vi "admin tables.vi"() -> ()   [LabVIEW 2020, in "Data.PG.lvclass"]
uses:
  Data.PG.lvclass
panel:
  out "path_to_selected_column":string="llab_038:d001(TEST_TABLE--new_stuff(hippos))"
  in  "Get path":bool
  out "table selected":string
  in  "max characters (if string)":i32
  in  "new column units":string="discoveries"
  in  "new column name":string="successfulness"
  in  "Create Column":bool
  in  "Ring":u16(ring) items=["double", "string", "integer", "boolean"]
  in  "columns_list":i32(listbox)=-1
  in  "new table name":string="TEST_TABLE_2"
  in  "Create Table":bool
  in  "tables_list":i32(listbox)=-1
  in  "STOP":bool
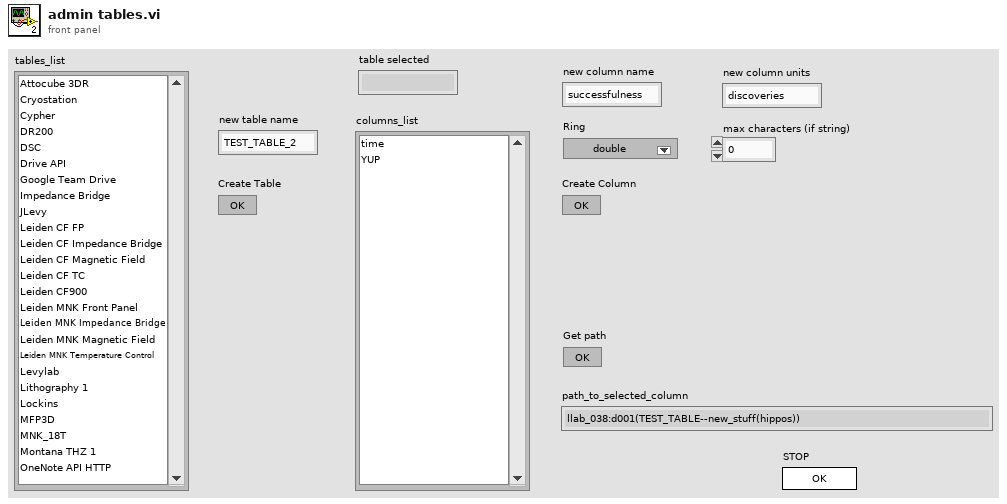
[diagram p1: front panel]
types:
  T1 = enum32{"Invalid", "Standard", "Closed", "Hidden", "Minimized", "Maximized"}
  T2 = enum32{"invalid app kind", "Development System", "Run Time System", "Student Edition", "Embedded LabVIEW", "Evaluation", "Custom"}
  T3 = cluster{"Core":cluster{"Current VI Reference":refnum<vi>, "Close Panel on Exit?":bool}, "Data.PG in":refnum<class "Data.PG.lvclass">, "connection info":cluster{"host":string, "port":string, "dbname":string, "user":string, "password":string}, "table names":string[], "table paths":string[], "column names":string[], "column units":string[], "column paths":string[], "new table name":string, "new column name":string, "new column data type":string, "new column units":string, "selected table":string, "selected column":string, "selected table path":string, "selected column path":string, "Start":timestamp, "End":timestamp, "max points":i32, "selected column units":string}
  T4 = cluster{"host":string, "port":string, "dbname":string, "user":string, "password":string}
  T5 = cluster{"Current VI Reference":refnum<vi>, "Close Panel on Exit?":bool}
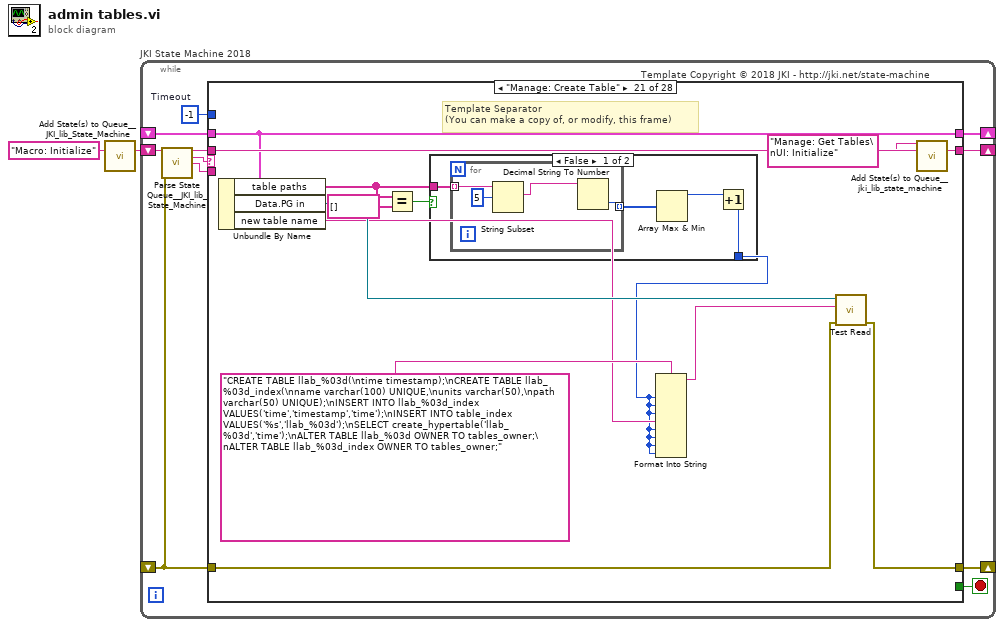
[diagram p0: block diagram]
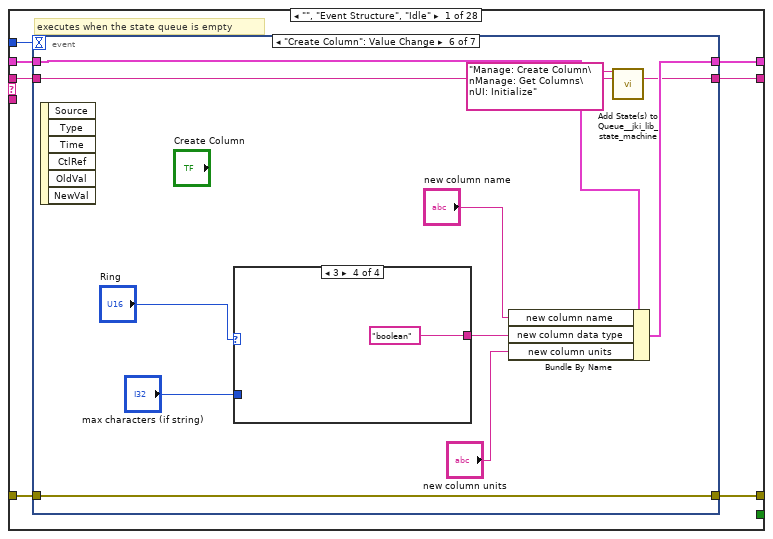
[diagram p2: hidden frame]
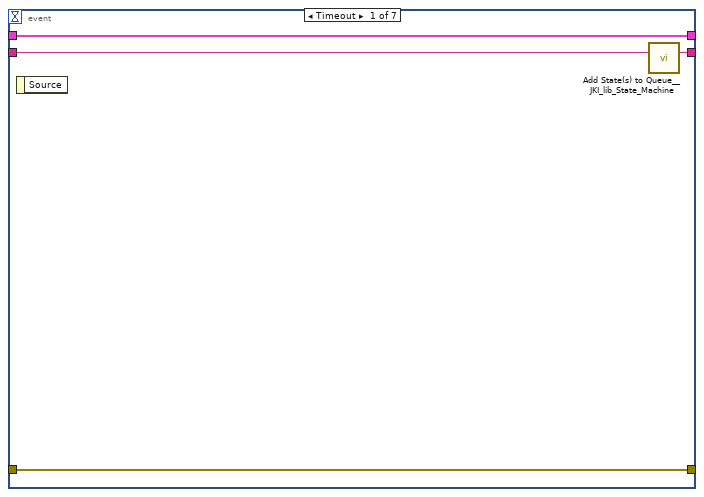
[diagram p3: hidden frame]
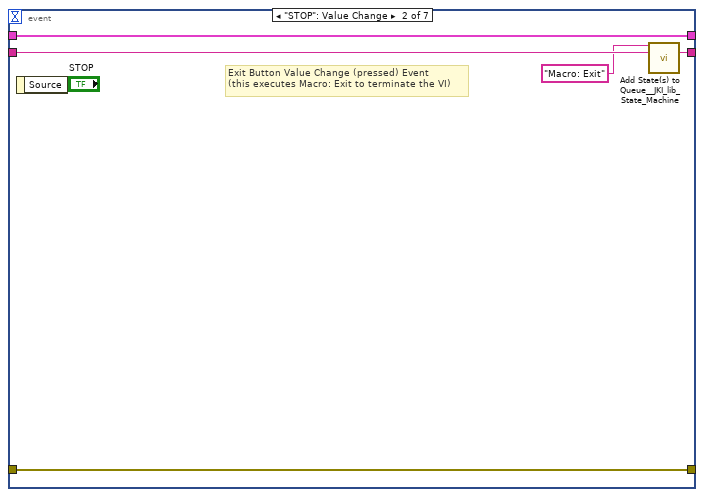
[diagram p4: hidden frame]
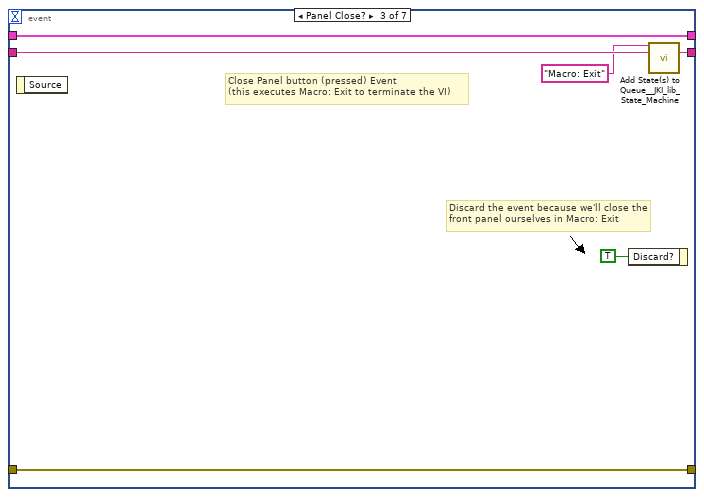
[diagram p5: hidden frame]
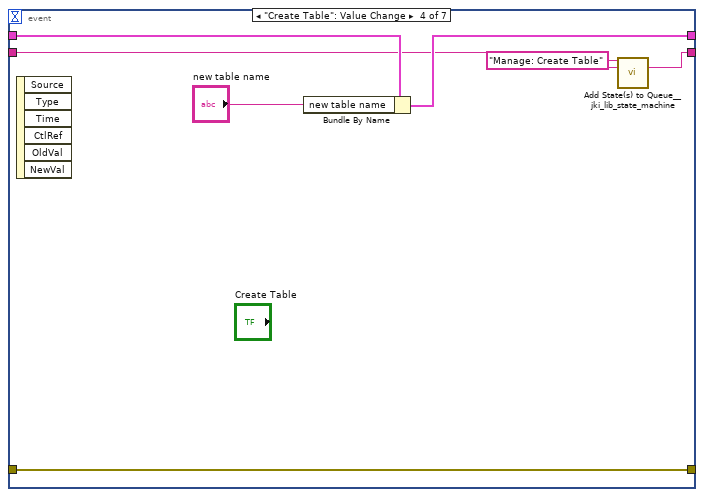
[diagram p6: hidden frame]
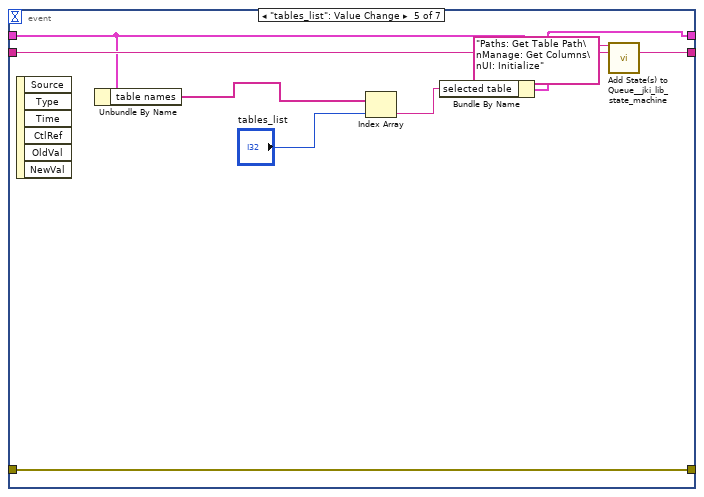
[diagram p7: hidden frame]
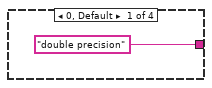
[diagram p8: hidden frame]
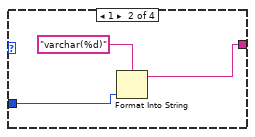
[diagram p9: hidden frame]
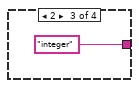
[diagram p10: hidden frame]
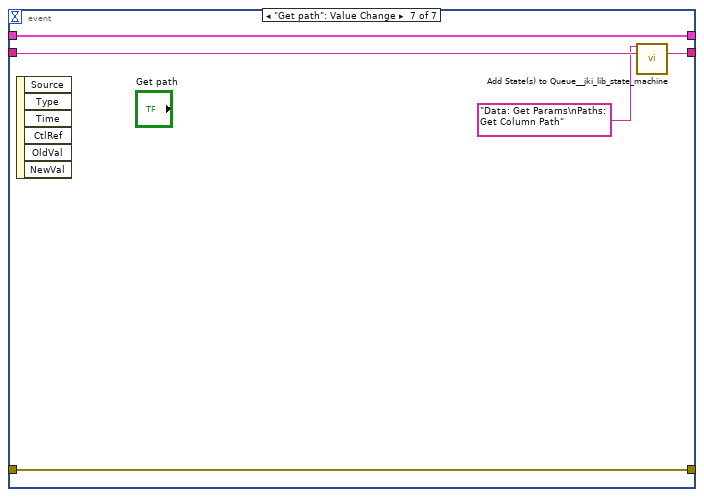
[diagram p11: hidden frame]
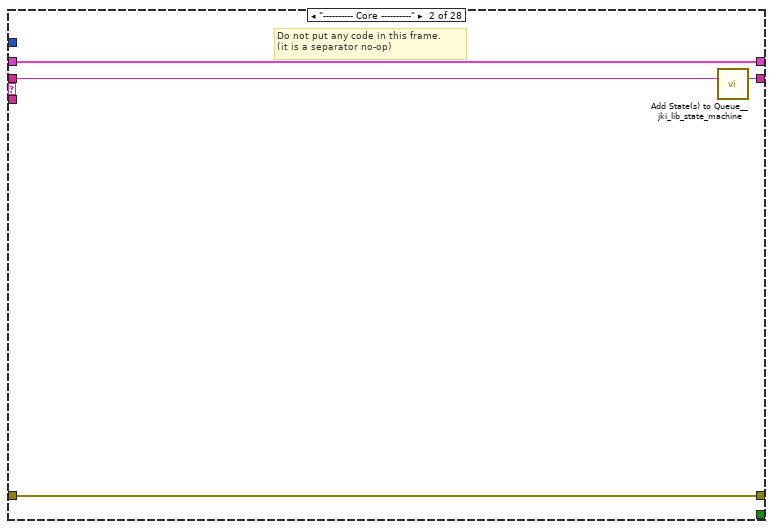
[diagram p12: hidden frame]
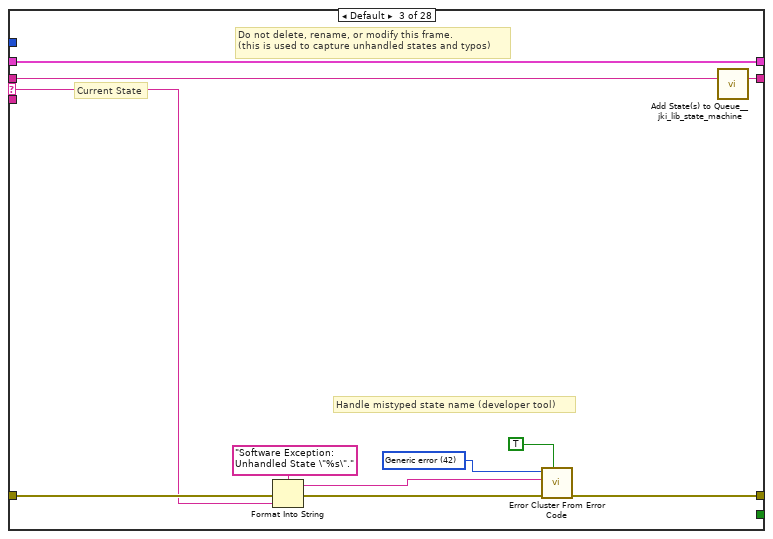
[diagram p13: hidden frame]
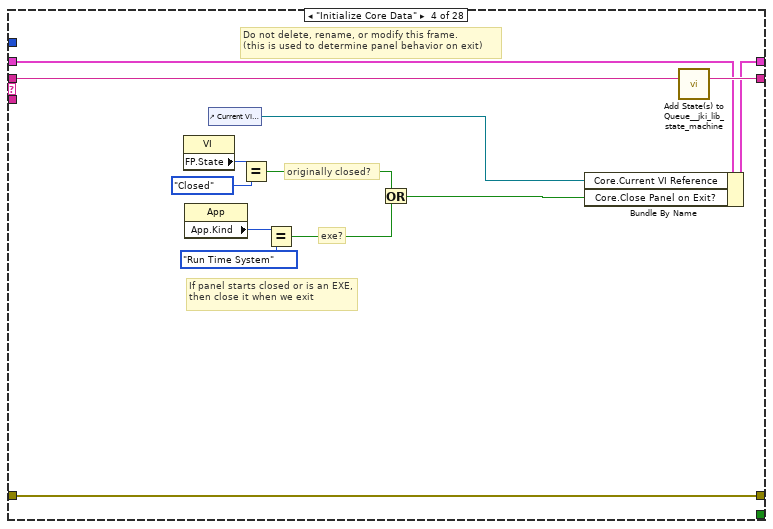
[diagram p14: hidden frame]
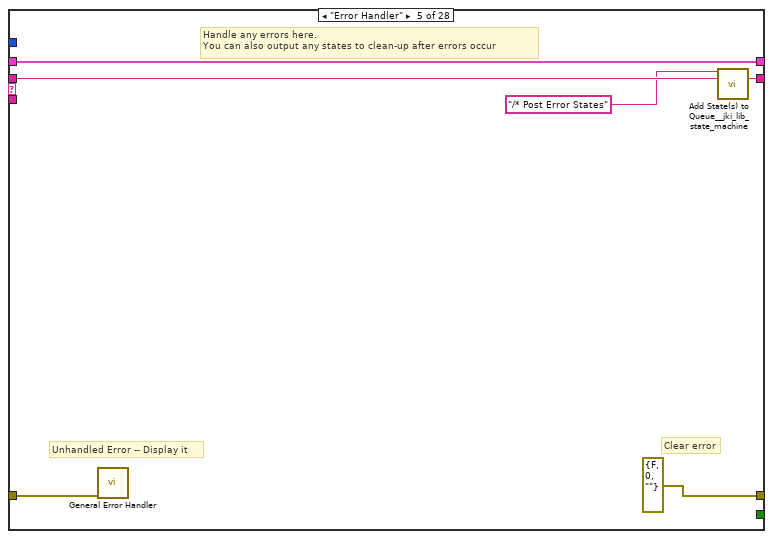
[diagram p15: hidden frame]
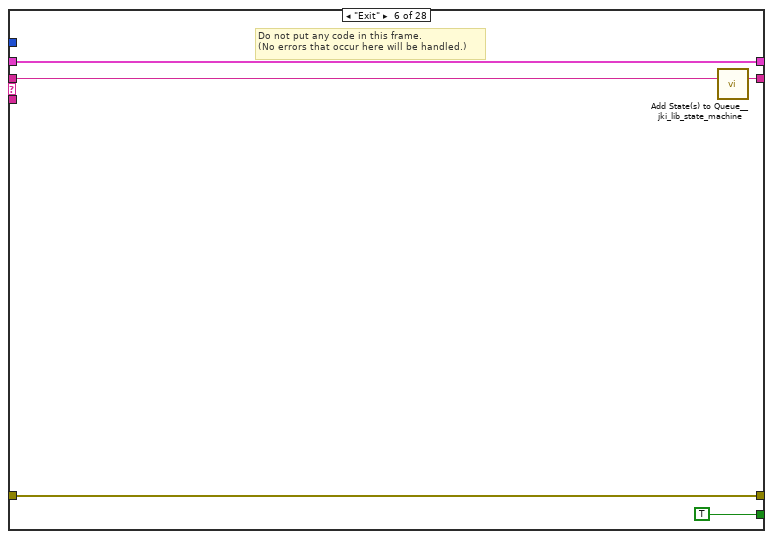
[diagram p16: hidden frame]
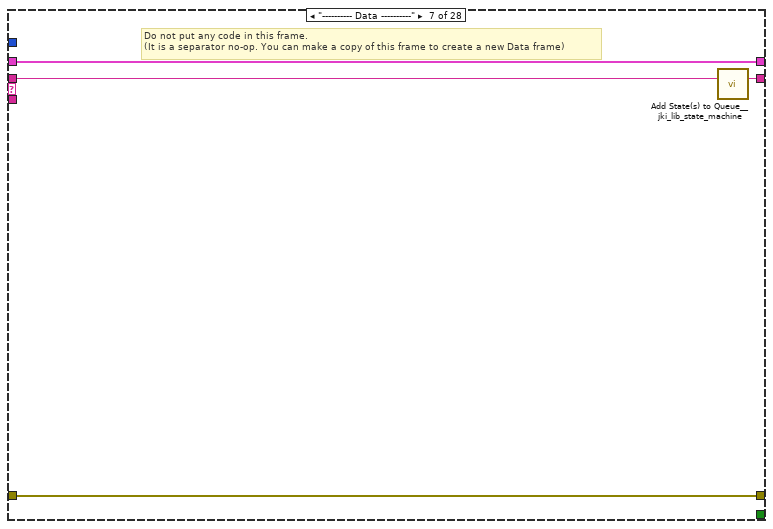
[diagram p17: hidden frame]
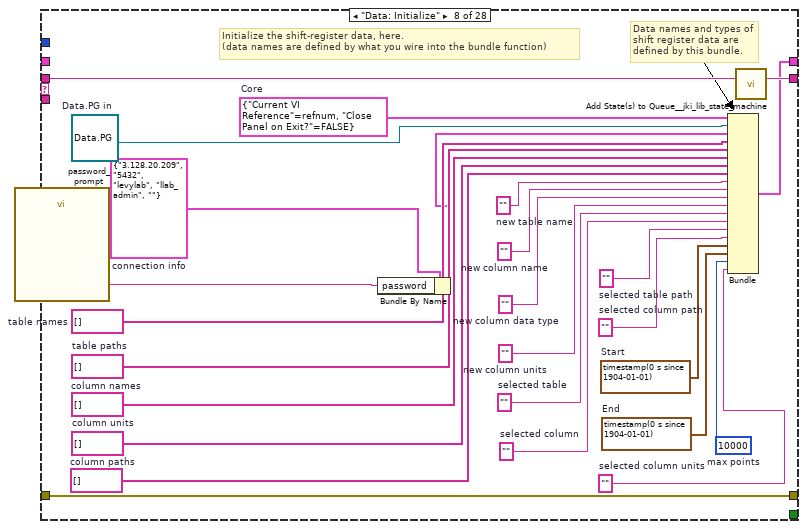
[diagram p18: hidden frame]
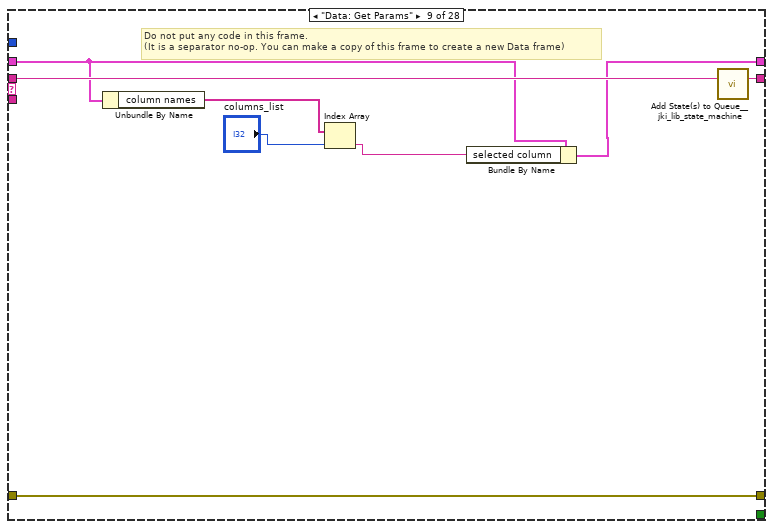
[diagram p19: hidden frame]
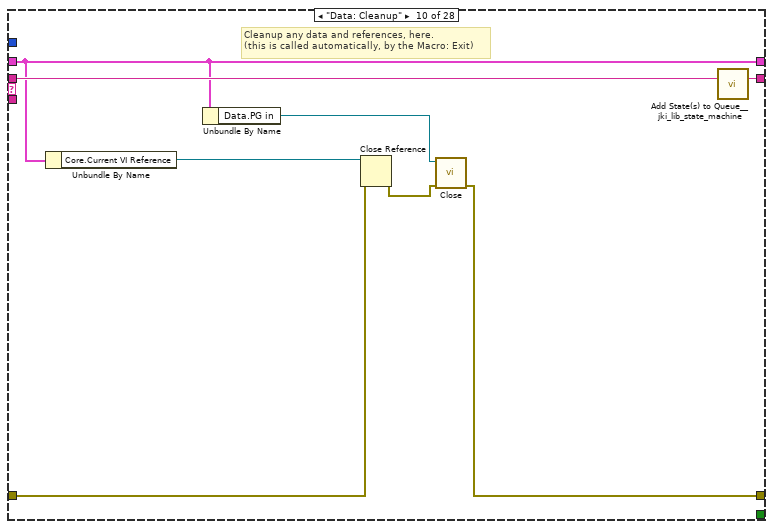
[diagram p20: hidden frame]
diagram:
  n1 = call <vilib>:"Add State(s) to Queue__JKI_lib_State_Machine.vi"("State(s) in (\"\")"="Macro: Initialize") -> ("States Out"=w2:string)  [unwired: 14 in]
  n2 = while "JKI State Machine 2018" {
    shift-right: [w6] -> _
    shift-left: _ -> [w5]
    shift-right: [w9] -> _
    shift-left: _ -> [w3]
    shift-right: [w8] -> _
    shift-left: w2 -> [w10]
    stop <- w7 stop-if-true
    w4 = -1  # Timeout
    # "Template Copyright © 2018 JKI - http://jki.net/state-machine"
    n3 = call <vilib>:"Parse State Queue__JKI_lib_State_Machine.vi"("State Queue"=w10, "Error In (no error)"=w3) -> ("Remaining States"=w12:string, "Current State"=w13:string, "Arguments"=w11:string)  [unwired: 11 in]
    n4 = case shown="\"Manage: Create Table\"" w13 {
      selector: w13 -> [_ _ w78 _ _ _ _ _ _ _ _ _ _ _ _ _ _ _ _ _ _ _ _ _ _ _ _ _]
      tunnel: w12 -> [w20 w77 w82 w101 w107 w112 w116 w142 w150 w158 w162 w169 w175 w186 w255 w260 w270 w274 w287 w306 w320 w354 w378 w384 w393 w397 w410 w414]
      tunnel: w11 -> [_ _ _ _ _ _ _ _ _ _ _ _ w170 w180 _ _ _ _ _ _ _ _ _ _ _ _ _ _]
      tunnel: w5 -> [w18 w74 w80 w94 w104 w110 w113 _ w146 w152 w159 w164 w173 w182 w252 w257 w267 w271 w279 w295 w318 w352 w375 w382 w387 w394 w402 w413]
      tunnel: [w17 w75 w84 w98 errorcluster {"status"=FALSE, "code"=0, "source"=""} ("error out") w109 w114 w139 w148 w153 w160 w167 w171 w183 w253 w258 w268 w272 w281 w289 w308 w338 w376 w379 w388 w395 w398 w411] -> w9
      tunnel: w3 -> [w16 w75 w83 w98 w103 w109 w114 w139 w148 w155 w160 w167 w172 w184 w253 w258 w268 w272 w282 w290 w309 w340 w376 w380 w389 w395 w399 w412]
      tunnel: [w19 w76 w81 w100 w106 w111 w115 w141 w149 w157 w161 w168 w174 w185 w254 w259 w269 w273 w286 w305 w319 w353 w377 w383 w392 w396 w409 w415] -> w8
      tunnel: [_ _ _ _ _ TRUE _ _ _ _ _ _ _ _ _ _ _ _ _ _ _ _ _ _ _ _ _ _] -> w7
      tunnel: [w15 w74 w80 w99 w104 w110 w113 w140 w147 w152 w159 w164 w173 w182 w252 w257 w267 w271 w278 w294 w318 w352 w375 w382 w386 w394 w401 w416] -> w6
      tunnel: w4 -> [w14 _ _ _ _ _ _ _ _ _ _ _ _ _ _ _ _ _ _ _ _ _ _ _ _ _ _ _]
      frame "", "Event Structure", "Idle" {
        # "executes when the state queue is empty"
        n5 = event shown="[5] \"Create Column\": Value Change" {
          selector: _ -> [_ _ _ _ _ _ _]
          dyn-events: _ -> [_ _ _ _ _ _ _]
          timeout: w14 -> [_ _ _ _ _ _ _]
          tunnel: w20 -> [w24 w29 w35 w38 w49 w53 w71]
          tunnel: [w23 w28 w34 w37 w50 w54 w72] -> w19
          tunnel: w18 -> [w21 w26 w32 w41 w45 w60 w73]
          tunnel: [w22 w27 w33 w42 w51 w55 w69] -> w17
          tunnel: w16 -> [w22 w27 w33 w42 w51 w55 w69]
          tunnel: [w21 w26 w32 w40 w44 w59 w73] -> w15
          event Timeout {
            n6 = event-data() -> ()  [unwired: 1 in, 1 out]
            n7 = call <vilib>:"Add State(s) to Queue__JKI_lib_State_Machine.vi"("State(s) in (\"\")"=w24) -> ("States Out"=w23:string)  [unwired: 14 in]
          }
          event "STOP": Value Change {
            # "Exit Button Value Change (pressed) Event\n(this executes Macro: Exit to terminate the VI)"
            n8 = event-data() -> ()  [unwired: 1 in, 1 out]
            n9 = call <vilib>:"Add State(s) to Queue__JKI_lib_State_Machine.vi"("State(s) in Front (\"\")"="Macro: Exit", "State(s) in (\"\")"=w29) -> ("States Out"=w28:string)  [unwired: 13 in]
          }
          event Panel Close? {
            # "Discard the event because we'll close the front panel ourselves in Macro: Exit"
            # "Close Panel button (pressed) Event\n(this executes Macro: Exit to terminate the VI)"
            n10 = event-data() -> ()  [unwired: 1 in, 1 out]
            n11 = event-data("Discard?"=TRUE) -> ()  [unwired: 1 in, 1 out]
            n12 = call <vilib>:"Add State(s) to Queue__JKI_lib_State_Machine.vi"("State(s) in Front (\"\")"="Macro: Exit", "State(s) in (\"\")"=w35) -> ("States Out"=w34:string)  [unwired: 13 in]
          }
          event "Create Table": Value Change {
            n13 = event-data() -> ()  [unwired: 1 in, 6 out]
            n14 = Bundle By Name(cluster=w41, "new table name"="new table name") -> (w40:T3)
            n15 = call <vilib>:"Add State(s) to Queue__jki_lib_state_machine.vi"("State(s) in Front (\"\")"="Manage: Create Table" ("State(s) in Front (\"\")"), "State(s) in (\"\")"=w38) -> ("States Out"=w37:string)  [unwired: 13 in]
          }
          event "tables_list": Value Change {
            n16 = event-data() -> ()  [unwired: 1 in, 6 out]
            n17 = Unbundle By Name(w45) -> ("table names"=w46:string[])
            n18 = Index Array(array=w46, index="tables_list") -> (element=w43:string)
            n19 = Bundle By Name(cluster=w45, "selected table"=w43) -> (w44:T3)
            n20 = call <vilib>:"Add State(s) to Queue__jki_lib_state_machine.vi"("State(s) in Front (\"\")"="Paths: Get Table Path\nManage: Get Columns\nUI: Initialize" ("State(s) in Front (\"\")"), "State(s) in (\"\")"=w49) -> ("States Out"=w50:string)  [unwired: 13 in]
          }
          event "Create Column": Value Change {
            n21 = event-data() -> ()  [unwired: 1 in, 6 out]
            n22 = case shown="3" "Ring" {
              tunnel: ["double precision" w64 "integer" "boolean"] -> w58
              tunnel: "max characters (if string)" -> [_ w65 _ _]
              frame 0, Default {
              }
              frame 1 {
                n23 = Format Into String(format string="varchar(%d)", w65) -> (resulting string=w64:string)  [unwired: 2 in, 1 out]
              }
              frame 2 {
              }
              frame 3 {
              }
            }
            n24 = Bundle By Name(cluster=w60, "new column name"="new column name", "new column data type"=w58, "new column units"="new column units") -> (w59:T3)
            n25 = call <vilib>:"Add State(s) to Queue__jki_lib_state_machine.vi"("State(s) in Front (\"\")"="Manage: Create Column\nManage: Get Columns\nUI: Initialize" ("State(s) in Front (\"\")"), "State(s) in (\"\")"=w53) -> ("States Out"=w54:string)  [unwired: 13 in]
          }
          event "Get path": Value Change {
            n26 = event-data() -> ()  [unwired: 1 in, 6 out]
            n27 = call <vilib>:"Add State(s) to Queue__jki_lib_state_machine.vi"("State(s) in Front (\"\")"="Data: Get Params\nPaths: Get Column Path", "State(s) in (\"\")"=w71) -> ("States Out"=w72:string)  [unwired: 13 in]
          }
        }
      }
      frame "---------- Core ----------" {
        # "Do not put any code in this frame.\n(it is a separator no-op)"
        n28 = call <vilib>:"Add State(s) to Queue__jki_lib_state_machine.vi"("State(s) in (\"\")"=w77) -> ("States Out"=w76:string)  [unwired: 14 in]
      }
      frame Default {
        w87 = 42 items=["No error", "Argument error", "Memory is full", "Out of zone", "End of file", "File already open", "Generic file I/O error", "File not found", "File permission error", "Disk is full", "Duplicate path", "Too many files open", "System feature not enabled", "Resource file not found", "Cannot add resource", "Resource not found", "Image not found", "Image memory error", "Pen does not exist", "Config type invalid", "Config token not found", "Config parse error", "Config memory error", "Bad external code format", "Bad external code offset", "External code not present", "Null window", "Destroy window error", "Null menu", "Print aborted", "Bad print record", "Print driver error", "Windows error during printing", "Memory error during printing", "Print dialog error", "Generic print error", "Invalid device refnum", "Device not found", "Device parameter error", "Device unit error", "Cannot open device", "Device call aborted", "Generic error", "Cancelled by user", "Object ID too low", "Object ID too high", "Object not in heap", "Unknown heap", "Unknown object (invalid DefProc)", "Unknown object (DefProc not in table)", "Message out of range", "Invalid (null) method", "Unknown message", "Manager call not supported", "Bad address", "Network operation in progress", "Network operation timed out", "Connection is busy", "Network attribute not supported", "Network error", "Address in use", "System out of memory", "Connection aborted", "Connection refused", "Not connected", "Already connected", "Connection closed", "Initialization error (interapplication manager)", "Bad occurrence", "Wait on unbound occurrence handler", "Occurrence queue overflow", "Datalog type conflict", "Unused", "Unrecognized type (interapplication manager)", "Memory corrupt", "Failed to make temporary DLL", "Old CIN version", "Drag socket not found", "Failed to load drop-object", "Failed to register OLE object", "Failed to release OLE object", "Format specifier type mismatch", "Unknown format specifier", "Too few format specifiers", "Too many format specifiers", "Scan failed", "Newer CIN version", "Error converting to variant", "Runtime menu error", "Password tampered", "Variant attribute not found", "Incompatible variant data type", "Event data is not available", "Event Store is not present", "Occurrence is not found", "Event Queue is not created", "Event info is not available", "Refnum passed is NULL", "Error retrieving Class GUID", "Error retrieving CoClass GUID", "Error retrieving TypeLib GUID.", "Bad built application magic bytes.", "Specific driver is different from the specific driver associated with the Logical Name.", "There is no session opened to the class driver.", "Max Error", "MAX - Error with config objects", "MAX - Error loading configuration", "MAX - Group not supported"]
        # "Current State"
        # "Do not delete, rename, or modify this frame.\n(this is used to capture unhandled states and typos)"
        # "Handle mistyped state name (developer tool)"
        n29 = Format Into String(format string="Software Exception: Unhandled State \"%s\"." ("message"), error in=w83, w78) -> (resulting string=w86:string, error out=w85:errorcluster)  [unwired: 1 in]
        n30 = call <vilib>:"Error Cluster From Error Code.vi"("show call chain? (False)"=TRUE, "error in (no error)"=w85, "error message (\"\")"=w86, "error code (0)"=w87) -> ("error out"=w84:errorcluster)  [unwired: 5 in]
        n31 = call <vilib>:"Add State(s) to Queue__jki_lib_state_machine.vi"("State(s) in (\"\")"=w82) -> ("States Out"=w81:string)  [unwired: 14 in]
      }
      frame "Initialize Core Data" {
        # "Do not delete, rename, or modify this frame.\n(this is used to determine panel behavior on exit)"
        # "originally closed?"
        # "exe?"
        # "If panel starts closed or is an EXE, then close it when we exit"
        n32 = property class="VI"() -> ("FP.State"=w91:T1)  [unwired: 2 in, 2 out]
        n33 = property class="App"() -> ("App.Kind"=w97:T2)  [unwired: 2 in, 2 out]
        n34 = control-ref of="Current VI Reference"() -> (w92:refnum<vi>)
        n35 = Equal?(x=w91, y=T1."Closed" ("Front Panel Window:State")) -> (x = y?=w89:bool)
        n36 = Equal?(x=w97, y=T2."Run Time System" ("Application:Kind")) -> (x = y?=w95:bool)
        n37 = Or(x=w89, y=w95) -> (x .or. y?=w93:bool)
        n38 = Bundle By Name(cluster=w94, "Core.Current VI Reference"=w92, "Core.Close Panel on Exit?"=w93) -> (w99:T3)
        n39 = call <vilib>:"Add State(s) to Queue__jki_lib_state_machine.vi"("State(s) in (\"\")"=w101) -> ("States Out"=w100:string)  [unwired: 14 in]
      }
      frame "Error Handler" {
        # "Unhandled Error -- Display it"
        # "Handle any errors here.\nYou can also output any states to clean-up after errors occur"
        # "Clear error"
        n40 = call <vilib>:"General Error Handler.vi"("error in (no error)"=w103) -> ()  [unwired: 10 in, 5 out]
        n41 = call <vilib>:"Add State(s) to Queue__jki_lib_state_machine.vi"("State(s) in Front (\"\")"="/* Post Error States", "State(s) in (\"\")"=w107) -> ("States Out"=w106:string)  [unwired: 13 in]
      }
      frame "Exit" {
        # "Do not put any code in this frame.\n(No errors that occur here will be handled.)"
        n42 = call <vilib>:"Add State(s) to Queue__jki_lib_state_machine.vi"("State(s) in (\"\")"=w112) -> ("States Out"=w111:string)  [unwired: 14 in]
      }
      frame "---------- Data ----------" {
        # "Do not put any code in this frame.\n(It is a separator no-op. You can make a copy of this frame to create a new Data frame)"
        n43 = call <vilib>:"Add State(s) to Queue__jki_lib_state_machine.vi"("State(s) in (\"\")"=w116) -> ("States Out"=w115:string)  [unwired: 14 in]
      }
      frame "Data: Initialize" {
        w120 = ""  # selected column units
        w121 = 10000  # max points
        w122 = timestamp(0 s since 1904-01-01)  # End
        w123 = timestamp(0 s since 1904-01-01)  # Start
        w124 = ""  # selected column path
        w125 = ""  # selected table path
        w126 = ""  # selected column
        w127 = ""  # selected table
        w128 = ""  # new column units
        w129 = ""  # new column data type
        w130 = ""  # new column name
        w131 = ""  # new table name
        w132 = string[] []  # column paths
        w133 = string[] []  # column units
        w134 = string[] []  # column names
        w135 = string[] []  # table paths
        w136 = string[] []  # table names
        w119 = T4 {"host"="3.128.20.209", "port"="5432", "dbname"="levylab", "user"="llab_admin", "password"=""}  # connection info
        w137 = refnum<class "Data.PG.lvclass"> refnum  # Data.PG in
        w138 = T5 {"Current VI Reference"=refnum, "Close Panel on Exit?"=FALSE}  # Core
        # "Data names and types of shift register data are defined by this bundle."
        # "Initialize the shift-register data, here.\n(data names are defined by what you wire into the bundle function)"
        n44 = call "password_prompt.vi"() -> ("password"=w117:string)  [unwired: 17 in, 2 out]
        n45 = Bundle By Name(cluster=w119, "password"=w117) -> (w118:T4)
        n46 = Bundle("Core"=w138, "Data.PG in"=w137, "connection info"=w118, "table names"=w136, "table paths"=w135, "column names"=w134, "column units"=w133, "column paths"=w132, "new table name"=w131, "new column name"=w130, "new column data type"=w129, "new column units"=w128, "selected table"=w127, "selected column"=w126, "selected table path"=w125, "selected column path"=w124, "Start"=w123, "End"=w122, "max points"=w121, "selected column units"=w120) -> (w140:T3)  [unwired: 1 in]
        n47 = call <vilib>:"Add State(s) to Queue__jki_lib_state_machine.vi"("State(s) in (\"\")"=w142) -> ("States Out"=w141:string)  [unwired: 14 in]
      }
      frame "Data: Get Params" {
        # "Do not put any code in this frame.\n(It is a separator no-op. You can make a copy of this frame to create a new Data frame)"
        n48 = Unbundle By Name(w146) -> ("column names"=w144:string[])
        n49 = Index Array(array=w144, index="columns_list") -> (element=w143:string)
        n50 = Bundle By Name(cluster=w146, "selected column"=w143) -> (w147:T3)
        n51 = call <vilib>:"Add State(s) to Queue__jki_lib_state_machine.vi"("State(s) in (\"\")"=w150) -> ("States Out"=w149:string)  [unwired: 14 in]
      }
      frame "Data: Cleanup" {
        # "Cleanup any data and references, here.\n(this is called automatically, by the Macro: Exit)"
        n52 = Unbundle By Name(w152) -> ("Core.Current VI Reference"=w156:refnum<vi>)
        n53 = Unbundle By Name(w152) -> ("Data.PG in"=w151:refnum<class "Data.PG.lvclass">)
        n54 = Close Reference(reference=w156, error in (no error)=w155) -> (error out=w154:errorcluster)
        n55 = call-dynamic "Close.vi"("error in (no error)"=w154, "Data.PG in"=w151) -> ("error out"=w153:errorcluster)  [unwired: 8 in, 1 out]
        n56 = call <vilib>:"Add State(s) to Queue__jki_lib_state_machine.vi"("State(s) in (\"\")"=w158) -> ("States Out"=w157:string)  [unwired: 14 in]
      }
      frame "---------- UI ----------" {
        # "Do not put any code in this frame.\n(It is a separator no-op. You can make a copy of this frame to create a new UI frame)"
        n57 = call <vilib>:"Add State(s) to Queue__jki_lib_state_machine.vi"("State(s) in (\"\")"=w162) -> ("States Out"=w161:string)  [unwired: 14 in]
      }
      frame "UI: Initialize" {
        # "Initialize the User Interface, here.\n(this is called automatically, by the Macro: Init)"
        n58 = Unbundle By Name(w164) -> ("table names"=w166:string[], "column names"=w165:string[], "selected table"=→"table selected":string)
        n59 = property on="tables_list" class="LstBox (strict)"("Item Names"=w166) -> ()  [unwired: 2 in, 2 out]
        n60 = property on="columns_list" class="LstBox (strict)"("Item Names"=w165) -> ()  [unwired: 2 in, 2 out]
        n61 = call <vilib>:"Add State(s) to Queue__jki_lib_state_machine.vi"("State(s) in (\"\")"=w169) -> ("States Out"=w168:string)  [unwired: 14 in]
      }
      frame "UI: Cursor Set" {
        # "Argument"
        # "Set and Unset Cursor Busy.\n(Usage: \"UI: Cursor Set >> Busy|Idle\")"
        n62 = case shown="\"Idle\", Default" w170 {
          tunnel: w172 -> [w177 w179]
          tunnel: [w176 w178] -> w171
          frame "Idle", Default {
            n63 = call <vilib>:"Unset Busy.vi"("error in (no error)"=w177) -> ("error out"=w176:errorcluster)  [unwired: 10 in]
          }
          frame "Busy" {
            n64 = call <vilib>:"Set Busy.vi"("error in (no error)"=w179) -> ("error out"=w178:errorcluster)  [unwired: 9 in, 1 out]
          }
        }
        n65 = call <vilib>:"Add State(s) to Queue__jki_lib_state_machine.vi"("State(s) in (\"\")"=w175) -> ("States Out"=w174:string)  [unwired: 14 in]
      }
      frame "UI: Front Panel State" {
        # "Argument"
        # "Set Front Panel Open or Closed\n(Usage: \"UI: Front Panel State >> Open|Close\")"
        n66 = Unbundle By Name(w182) -> ("Core.Current VI Reference"=w181:refnum<vi>)
        n67 = case shown="\"Minimize\", \"Minimized\"" w180 {
          tunnel: w184 -> [w192 w207 w218 w231 w244]
          tunnel: [w194 w208 w220 w233 w246] -> w183
          tunnel: w181 -> [w193 w205 w219 w232 w245]
          frame "Open", "Standard", Default {
            w187 = T1."Standard" ("State")
            n68 = property class="VI"(reference=w193, error in=w192) -> (reference out=w190:refnum<vi>, error out=w191:errorcluster, "FP.State"=w189:T1)
            n69 = Not Equal?(x=w189, y=w187) -> (x != y?=w188:bool)
            n70 = case shown="True" w188 {
              tunnel: [w198 w200] -> w194
              tunnel: w191 -> [w197 w200]
              tunnel: w190 -> [w196 _]
              tunnel: w187 -> [w195 _]
              frame True {
                n71 = invoke class="VI" method="FP.Open"(reference=w196, error in=w197, "Activate"=TRUE, "State"=w195) -> (error out=w198:errorcluster)  [unwired: 1 in, 4 out]
              }
              frame False {
              }
            }
          }
          frame "Close", "Closed" {
            n72 = property class="VI"(reference=w205, error in=w207) -> (reference out=w204:refnum<vi>, error out=w206:errorcluster, "FP.State"=w202:T1)
            n73 = Not Equal?(x=w202, y=T1."Closed" ("Front Panel Window:State")) -> (x != y?=w201:bool)
            n74 = case shown="True" w201 {
              tunnel: [w209 w212] -> w208
              tunnel: w206 -> [w209 w211]
              tunnel: w204 -> [_ w210]
              frame False {
              }
              frame True {
                n75 = invoke class="VI" method="FP.Close"(reference=w210, error in=w211) -> (error out=w212:errorcluster)  [unwired: 1 in, 2 out]
              }
            }
          }
          frame "Hidden", "Hide" {
            w213 = T1."Hidden" ("State")
            n76 = property class="VI"(reference=w219, error in=w218) -> (reference out=w216:refnum<vi>, error out=w217:errorcluster, "FP.State"=w215:T1)
            n77 = Not Equal?(x=w215, y=w213) -> (x != y?=w214:bool)
            n78 = case shown="True" w214 {
              tunnel: [w224 w225] -> w220
              tunnel: w217 -> [w223 w225]
              tunnel: w216 -> [w222 _]
              tunnel: w213 -> [w221 _]
              frame True {
                n79 = invoke class="VI" method="FP.Open"(reference=w222, error in=w223, "State"=w221) -> (error out=w224:errorcluster)  [unwired: 2 in, 4 out]
              }
              frame False {
              }
            }
          }
          frame "Minimize", "Minimized" {
            w226 = T1."Minimized" ("State")
            n80 = property class="VI"(reference=w232, error in=w231) -> (reference out=w229:refnum<vi>, error out=w230:errorcluster, "FP.State"=w228:T1)
            n81 = Not Equal?(x=w228, y=w226) -> (x != y?=w227:bool)
            n82 = case shown="True" w227 {
              tunnel: [w237 w238] -> w233
              tunnel: w230 -> [w236 w238]
              tunnel: w229 -> [w235 _]
              tunnel: w226 -> [w234 _]
              frame True {
                n83 = invoke class="VI" method="FP.Open"(reference=w235, error in=w236, "State"=w234) -> (error out=w237:errorcluster)  [unwired: 2 in, 4 out]
              }
              frame False {
              }
            }
          }
          frame "Maximize", "Maximized" {
            w239 = T1."Maximized" ("State")
            n84 = property class="VI"(reference=w245, error in=w244) -> (reference out=w242:refnum<vi>, error out=w243:errorcluster, "FP.State"=w241:T1)
            n85 = Not Equal?(x=w241, y=w239) -> (x != y?=w240:bool)
            n86 = case shown="True" w240 {
              tunnel: [w250 w251] -> w246
              tunnel: w243 -> [w249 w251]
              tunnel: w242 -> [w248 _]
              tunnel: w239 -> [w247 _]
              frame True {
                n87 = invoke class="VI" method="FP.Open"(reference=w248, error in=w249, "State"=w247) -> (error out=w250:errorcluster)  [unwired: 2 in, 4 out]
              }
              frame False {
              }
            }
          }
        }
        n88 = call <vilib>:"Add State(s) to Queue__jki_lib_state_machine.vi"("State(s) in (\"\")"=w186) -> ("States Out"=w185:string)  [unwired: 14 in]
      }
      frame "---------- Macro ----------" {
        # "Do not put any code in this frame.\n(It is a separator no-op. You can make a copy of this frame to create a new Macro frame)"
        n89 = call <vilib>:"Add State(s) to Queue__jki_lib_state_machine.vi"("State(s) in (\"\")"=w255) -> ("States Out"=w254:string)  [unwired: 14 in]
      }
      frame "Macro: Initialize" {
        w256 = "Data: Initialize\nInitialize Core Data\nConnection: Open\nManage: Get Tables\nUI: Initialize\nUI: Front Panel State >> Open"  # Data: Initialize Initialize Core Data Connection: Open Manage: Get Tables UI: Initialize UI: Front Panel State >> Open
        # "Initialization Macro\n(This is called once, when the VI starts)"
        n90 = call <vilib>:"Add State(s) to Queue__jki_lib_state_machine.vi"("State(s) in Front (\"\")"=w256, "State(s) in (\"\")"=w260) -> ("States Out"=w259:string)  [unwired: 13 in]
      }
      frame "Macro: Exit" {
        # "Exit Macro\n(This is called once, when the VI exits)"
        n91 = Unbundle By Name(w267) -> ("Core.Close Panel on Exit?"=w266:bool)
        n92 = Select(t="UI: Front Panel State >> Close", s=w266, f="") -> (s? t:f=w263:string)
        n93 = call <vilib>:"Add State(s) to Queue__jki_lib_state_machine.vi"("State(s) in (\"\")"=w263, "State(s) at Back (\"\")"="Data: Cleanup\nConnection: Close\nExit") -> ("States Out"=w261:string)  [unwired: 13 in]
        n94 = call <vilib>:"Add State(s) to Queue__jki_lib_state_machine.vi"("State(s) in Front (\"\")"=w261, "State(s) in (\"\")"=w270) -> ("States Out"=w269:string)  [unwired: 13 in]
      }
      frame "---------- Manage ----------" {
        # "Template Separator\n(You can make a copy of, or modify, this frame)"
        n95 = call <vilib>:"Add State(s) to Queue__jki_lib_state_machine.vi"("State(s) in (\"\")"=w274) -> ("States Out"=w273:string)  [unwired: 14 in]
      }
      frame "Manage: Get Tables" {
        # "Your code here.\n(You can make a copy of, or modify, this frame)"
        n96 = Unbundle By Name(w279) -> ("Data.PG in"=w285:refnum<class "Data.PG.lvclass">)
        n97 = call-dynamic "Test Read.vi"("error in (no error)"=w282, "command"="SELECT * FROM table_index ORDER BY name;", "Data.PG in"=w285) -> ("error out"=w281:errorcluster, "Result"=w283:string[][])  [unwired: 3 in, 4 out]
        n98 = Transpose 2D Array(2D array=w283) -> (transposed array=w280:string[][])
        n99 = Index Array(array=w280, index (row) #2=1 ("index (row)")) -> (element #1=w277:string[], element #2=w275:string[])  [unwired: 3 in]
        n100 = Bundle By Name(cluster=w279, "table names"=w277, "table paths"=w275) -> (w278:T3)
        n101 = call <vilib>:"Add State(s) to Queue__jki_lib_state_machine.vi"("State(s) in (\"\")"=w287) -> ("States Out"=w286:string)  [unwired: 14 in]
      }
      frame "Manage: Get Columns" {
        # "Your code here.\n(You can make a copy of, or modify, this frame)"
        n102 = Unbundle By Name(w295) -> ("Data.PG in"=w304:refnum<class "Data.PG.lvclass">, "selected table path"=w302:string)
        n103 = Format Into String(format string="SELECT * FROM %s_index; ", w302) -> (resulting string=w301:string)  [unwired: 2 in, 1 out]
        n104 = call-dynamic "Test Read.vi"("error in (no error)"=w290, "command"=w301, "Data.PG in"=w304) -> ("error out"=w289:errorcluster, "Result"=w300:string[][])  [unwired: 3 in, 4 out]
        n105 = Transpose 2D Array(2D array=w300) -> (transposed array=w299:string[][])
        n106 = Index Array(array=w299, index (row) #1=0 ("index (row)"), index (row) #2=1 ("index (row)"), index (row) #3=2 ("index (row)")) -> (element #1=w293:string[], element #2=w292:string[], element #3=w291:string[])  [unwired: 3 in]
        n107 = Bundle By Name(cluster=w295, "column names"=w293, "column units"=w292, "column paths"=w291) -> (w294:T3)
        n108 = call <vilib>:"Add State(s) to Queue__jki_lib_state_machine.vi"("State(s) in Front (\"\")"="UI: Initialize" ("State(s) in Front (\"\")"), "State(s) in (\"\")"=w306) -> ("States Out"=w305:string)  [unwired: 13 in]
      }
      frame "Manage: Create Table" {
        # "Template Separator\n(You can make a copy of, or modify, this frame)"
        n109 = Unbundle By Name(w318) -> ("table paths"=w311:string[], "Data.PG in"=w317:refnum<class "Data.PG.lvclass">, "new table name"=w314:string)
        n110 = Equal?(x=w311, y=string[] []) -> (x = y?=w312:bool)
        n111 = case shown="False" w312 {
          tunnel: w311 -> [w324 _]
          tunnel: [w321 0] -> w307
          frame False {
            n112 = for {
              tunnel: w324 -> [w328] mode=indexing
              tunnel: [w325] -> w323 mode=indexing
              n113 = String Subset(string=w328, offset (0)=5) -> (substring=w326:string)  [unwired: 1 in]
              n114 = Decimal String To Number(string=w326) -> (number=w325:i32)  [unwired: 2 in, 1 out]
            }
            n115 = Array Max & Min(array=w323) -> (max value=w322:i32)  [unwired: 3 out]
            n116 = Increment(x=w322) -> (x+1=w321:i32)
          }
          frame True {
          }
        }
        n117 = Format Into String(format string="CREATE TABLE llab_%03d(\ntime timestamp);\nCREATE TABLE llab_%03d_index(\nname varchar(100) UNIQUE,\nunits varchar(50),\npath varchar(50) UNIQUE);\nINSERT INTO llab_%03d_index VALUES('time','timestamp','time');\nINSERT INTO table_index VALUES('%s','llab_%03d');\nSELECT create_hypertable('llab_%03d','time');\nALTER TABLE llab_%03d OWNER TO tables_owner;\nALTER TABLE llab_%03d_index OWNER TO tables_owner;", w307, w307, w307, w314, w307, w307, w307, w307) -> (resulting string=w315:string)  [unwired: 2 in, 1 out]
        n118 = call-dynamic "Test Read.vi"("error in (no error)"=w309, "command"=w315, "Data.PG in"=w317) -> ("error out"=w308:errorcluster)  [unwired: 3 in, 5 out]
        n119 = call <vilib>:"Add State(s) to Queue__jki_lib_state_machine.vi"("State(s) in Front (\"\")"="Manage: Get Tables\nUI: Initialize" ("State(s) in Front (\"\")"), "State(s) in (\"\")"=w320) -> ("States Out"=w319:string)  [unwired: 13 in]
      }
      frame "Manage: Create Column" {
        # "Template Separator\n(You can make a copy of, or modify, this frame)"
        n120 = Unbundle By Name(w352) -> ("Data.PG in"=w346:refnum<class "Data.PG.lvclass">, "selected table path"=w334:string, "new column data type"=w335:string, "new column name"=w333:string, "new column units"=w332:string)
        n121 = String Subset(string=w335, length (rest)=1 ("length (rest)")) -> (substring=w348:string)  [unwired: 1 in]
        n122 = Equal?(x=w348, y="\"v\"") -> (x = y?=w349:bool)
        n123 = case shown="True" w349 {
          tunnel: w348 -> [w373 _]
          tunnel: [w373 "s"] -> w331
          frame False {
          }
          frame True {
          }
        }
        n124 = Format Into String(format string="SELECT column_name FROM information_schema.columns WHERE table_name = '%s' AND column_name LIKE '%s%%'", w334, w331) -> (resulting string=w345:string)  [unwired: 2 in, 1 out]
        n125 = call-dynamic "Test Read.vi"("error in (no error)"=w340, "command"=w345, "Data.PG in"=w346) -> ("error out"=w339:errorcluster, "Data.PG out"=w341:refnum<class "Data.PG.lvclass">, "Result"=w344:string[][])  [unwired: 3 in, 3 out]
        n126 = Equal?(x=w344, y=string[][] [] ("Result")) -> (x = y?=w342:bool)
        n127 = case shown="True" w342 {
          tunnel: w344 -> [w357 _]
          tunnel: [w355 0] -> w330
          frame False {
            n128 = Transpose 2D Array(2D array=w357) -> (transposed array=w367:string[][])
            n129 = Index Array(array=w367) -> (element=w360:string[])  [unwired: 2 in]
            n130 = Index Array(array=w360) -> (element=w366:string)  [unwired: 1 in]
            n131 = Equal?(x=w366, y="time") -> (x = y?=w364:bool)
            n132 = Select(t=1.0, s=w364, f=0.0) -> (s? t:f=w363:dbl)
            n133 = Array Subset(array=w360, index=w363) -> (w359:string[])  [unwired: 1 in]
            n134 = for {
              tunnel: w359 -> [w371] mode=indexing
              tunnel: [w368] -> w358 mode=indexing
              n135 = String Subset(string=w371, offset (0)=1) -> (substring=w369:string)  [unwired: 1 in]
              n136 = Decimal String To Number(string=w369) -> (number=w368:i32)  [unwired: 2 in, 1 out]
            }
            n137 = Array Max & Min(array=w358) -> (max value=w356:i32)  [unwired: 3 out]
            n138 = Increment(x=w356) -> (x+1=w355:i32)
          }
          frame True {
          }
        }
        n139 = Format Into String(format string="ALTER TABLE %s ADD COLUMN %s%03d %s;\nINSERT INTO %s_index VALUES('%s','%s','%s%03d');", w334, w331, w330, w335, w334, w333, w332, w331, w330) -> (resulting string=w337:string)  [unwired: 2 in, 1 out]
        n140 = call-dynamic "Test Read.vi"("error in (no error)"=w339, "command"=w337, "Data.PG in"=w341) -> ("error out"=w338:errorcluster)  [unwired: 3 in, 5 out]
        n141 = call <vilib>:"Add State(s) to Queue__jki_lib_state_machine.vi"("State(s) in (\"\")"=w354) -> ("States Out"=w353:string)  [unwired: 14 in]
      }
      frame "---------- Connection ----------" {
        # "Template Separator\n(You can make a copy of, or modify, this frame)"
        n142 = call <vilib>:"Add State(s) to Queue__jki_lib_state_machine.vi"("State(s) in (\"\")"=w378) -> ("States Out"=w377:string)  [unwired: 14 in]
      }
      frame "Connection: Close" {
        # "Template Separator\n(You can make a copy of, or modify, this frame)"
        n143 = Unbundle By Name(w382) -> ("Data.PG in"=w381:refnum<class "Data.PG.lvclass">)
        n144 = call-dynamic "Close.vi"("error in (no error)"=w380, "Data.PG in"=w381) -> ("error out"=w379:errorcluster)  [unwired: 8 in, 1 out]
        n145 = call <vilib>:"Add State(s) to Queue__jki_lib_state_machine.vi"("State(s) in (\"\")"=w384) -> ("States Out"=w383:string)  [unwired: 14 in]
      }
      frame "Connection: Open" {
        # "Template Separator\n(You can make a copy of, or modify, this frame)"
        n146 = Unbundle By Name(w387) -> ("Data.PG in"=w391:refnum<class "Data.PG.lvclass">, "connection info"=w390:T4)
        n147 = call "Set Connection Info.vi"("error in (no error)"=w389, "connection info"=w390, "Data.PG in"=w391) -> ("error out"=w388:errorcluster, "Data.PG out"=w385:refnum<class "Data.PG.lvclass">)  [unwired: 7 in]
        n148 = Bundle By Name(cluster=w387, "Data.PG in"=w385) -> (w386:T3)
        n149 = call <vilib>:"Add State(s) to Queue__jki_lib_state_machine.vi"("State(s) in (\"\")"=w393) -> ("States Out"=w392:string)  [unwired: 14 in]
      }
      frame "---------- Paths ----------" {
        # "Template Separator\n(You can make a copy of, or modify, this frame)"
        n150 = call <vilib>:"Add State(s) to Queue__jki_lib_state_machine.vi"("State(s) in (\"\")"=w397) -> ("States Out"=w396:string)  [unwired: 14 in]
      }
      frame "Paths: Get Table Path" {
        # "Template Separator\n(You can make a copy of, or modify, this frame)"
        n151 = Unbundle By Name(w402) -> ("Data.PG in"=w407:refnum<class "Data.PG.lvclass">, "selected table"=w405:string)
        n152 = Format Into String(format string="SELECT path FROM table_index WHERE name='%s'", w405) -> (resulting string=w406:string)  [unwired: 2 in, 1 out]
        n153 = call-dynamic "Test Read.vi"("error in (no error)"=w399, "command"=w406, "Data.PG in"=w407) -> ("error out"=w398:errorcluster, "Result"=w404:string[][])  [unwired: 3 in, 4 out]
        n154 = Index Array(array=w404) -> (element=w403:string[])  [unwired: 2 in]
        n155 = Index Array(array=w403) -> (element=w400:string)  [unwired: 1 in]
        n156 = Bundle By Name(cluster=w402, "selected table path"=w400) -> (w401:T3)
        n157 = call <vilib>:"Add State(s) to Queue__jki_lib_state_machine.vi"("State(s) in (\"\")"=w410) -> ("States Out"=w409:string)  [unwired: 14 in]
      }
      frame "Paths: Get Column Path" {
        # "Template Separator\n(You can make a copy of, or modify, this frame)"
        n158 = Unbundle By Name(w413) -> ("Data.PG in"=w434:refnum<class "Data.PG.lvclass">, "selected table path"=w427:string, "selected column"=w430:string, "selected table"=w422:string, "selected column"=w420:string)
        n159 = Format Into String(format string="SELECT path,units FROM %s_index WHERE name='%s'", w427, w430) -> (resulting string=w433:string)  [unwired: 2 in, 1 out]
        n160 = call-dynamic "Test Read.vi"("error in (no error)"=w412, "command"=w433, "Data.PG in"=w434) -> ("error out"=w411:errorcluster, "Result"=w432:string[][])  [unwired: 3 in, 4 out]
        n161 = Index Array(array=w432) -> (element=w431:string[])  [unwired: 2 in]
        n162 = Index Array(array=w431, index #1=0 ("index"), index #2=1 ("index")) -> (element #1=w425:string, element #2=w418:string)
        n163 = Bundle By Name(cluster=w413, "selected column path"=w425, "selected column units"=w418) -> (w416:T3)
        n164 = Concatenate Strings(w427, ":" ("string"), w425, "(" ("string"), w422, "--" ("string"), w420, "(" ("string"), w418, "))" ("string")) -> (→"path_to_selected_column":string)
        n165 = call <vilib>:"Add State(s) to Queue__jki_lib_state_machine.vi"("State(s) in (\"\")"=w414) -> ("States Out"=w415:string)  [unwired: 14 in]
      }
    }
  }
